vi "Send Read and Send Configuration.vi"(7 "Message Priority (Normal)":T3=enum."Normal", 8 "error in (no error)":errorcluster, 9 "Intrs":T1, 10 "Excitation":T2, 11 "Message Enqueuer":refnum<class "Message Enqueuer.lvclass">) -> (0 "error out":errorcluster, 3 "Message Enqueuer out":refnum<class "Message Enqueuer.lvclass">)   [LabVIEW 2023, in "MSS Host Actor.lvlib" / "Read and Send Configuration Msg.lvclass"]
doc: "This VI sends the message to an actor."
uses:
  Read and Send Configuration Msg.lvclass
  <vilib>/ActorFramework/Message Enqueuer/Message Enqueuer.lvclass
  <vilib>/ActorFramework/Message Enqueuer/Message Priority.ctl
  C:/Program Files/National Instruments/LabVIEW 2023/vi.lib/ActorFramework/Message/Message.lvclass
  Read and Send Configuration Msg.lvclass/Read and Send Configuration Msg.ctl
  <vilib>/ActorFramework/Message Enqueuer/Message Enqueuer.lvclass/Message Enqueuer.ctl
  <vilib>/Utility/LVClass/Get LV Class Name.vi
  <resource>/AFDebug/Generate Trace for Message.vi
  <vilib>/ActorFramework/Message Priority Queue/Priority Enqueue.vi
  D:/git/HAL/MSS/MSS Host Actor Messages/Read and Send Configuration Msg/Read and Send Configuration Msg.lvclass
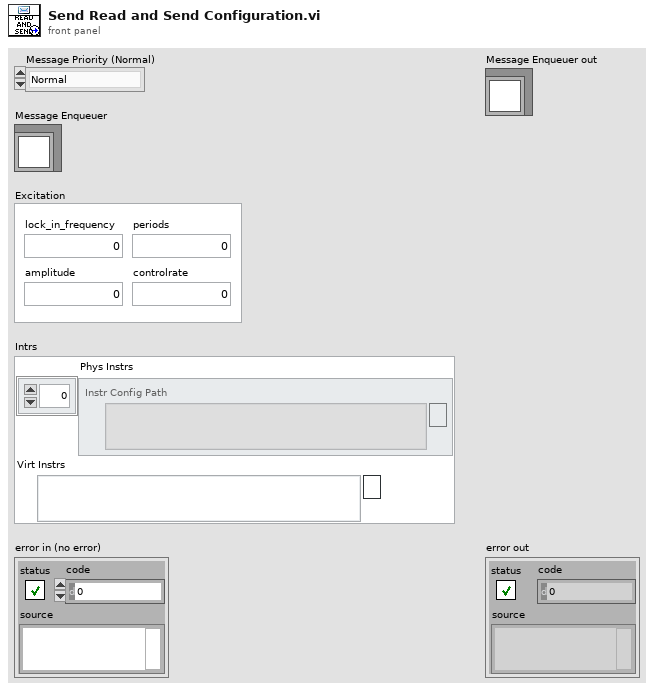
[diagram p1: front panel]
types:
  T1 = cluster{"Phys Instrs":path[], "Virt Instrs":path}
  T2 = cluster{"lock_in_frequency":dbl, "amplitude":dbl, "periods":dbl, "controlrate":dbl}
  T3 = typedef "Actor Framework.lvlib/Message Enqueuer.lvclass/Message Priority.ctl" = enum16{"Low", "Normal", "High"}
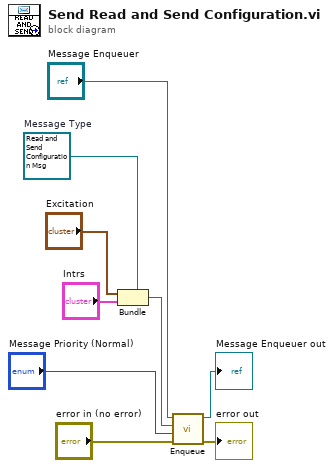
[diagram p0: block diagram]
diagram:
  w6 = refnum<class "Read and Send Configuration Msg.lvclass"> refnum  # Message Type
  n1 = Bundle(cluster=w6, "Excitation", "Intrs") -> (w5:refnum<class "Read and Send Configuration Msg.lvclass">)
  n2 = call <vilib>:"Enqueue.vi"("error in (no error)"="error in (no error)", "Message Priority (Normal)"="Message Priority (Normal)", "Message"=w5, "Message Enqueuer in"="Message Enqueuer") -> ("error out"=→"error out":errorcluster, "Message Enqueuer in"=→"Message Enqueuer out":refnum<class "Message Enqueuer.lvclass">)  [unwired: 6 in]
